vi "Read Data.vi"(8 "error in (no error)":errorcluster caption="entrée d'erreur (pas d'erreur)", 11 "Database Altyor en entrée":refnum<class "Database Altyor.lvclass">) -> (0 "error out":errorcluster caption="sortie d'erreur", 3 "Database Altyor en sortie":refnum<class "Database Altyor.lvclass">)   [LabVIEW 2020, in "Library Instrument & Equipement.lvlib" / "Library Database.lvlib" / "Database Altyor.lvclass"]
uses:
  Database Altyor.lvclass
  C:/Users/ngarcin/OneDrive - Altyor/Standard TB/Class/Database/Database drivers/Database Drivers.lvclass
  <vilib>/addons/database/_DB Variant To Data/Database Variant To Data.xnode
  Database Altyor.lvclass/Database Altyor.ctl
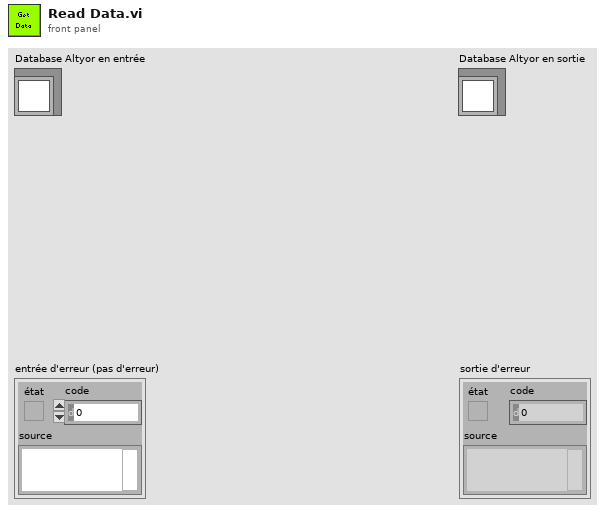
[diagram p1: front panel]
types:
  T1 = cluster{"idTest":u32, "CreationDate":string, "EndOfProduction":string, "OrderNumber":string, "Batch":string, "ProductName":string, "PartNumber":string, "SerialNumber":string, "Operator":string, "Result":string, "AdditionalInformation":string}[]
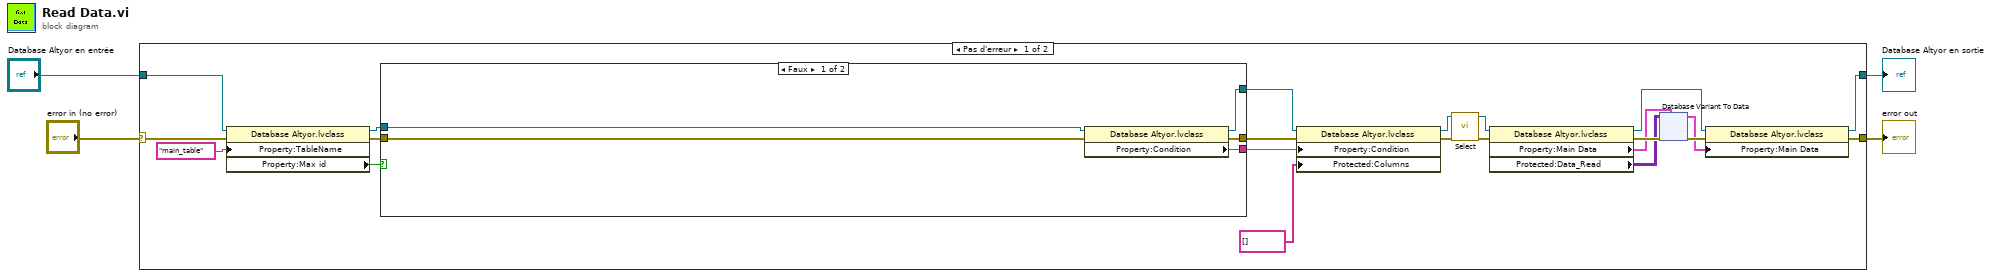
[diagram p0: block diagram]
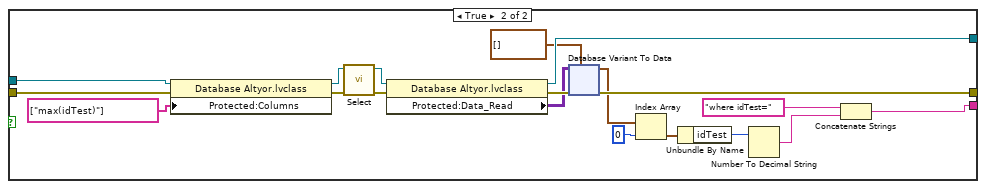
[diagram p2: hidden frame]
diagram:
  n1 = case shown="Pas d'erreur" "error in (no error)" {
    selector: "error in (no error)" -> [w13 w444]
    tunnel: [w22 w444] -> w3
    tunnel: [w20 w443] -> w1
    tunnel: "Database Altyor en entrée" -> [w14 w443]
    frame No Error {
      n2 = property class="Database Altyor.lvclass"(reference=w14, error in=w13, "Property:TableName"="main_table" ("TableName")) -> (reference out=w8:refnum<class "Database Altyor.lvclass">, error out=w10:errorcluster, "Property:Max id"=w11:bool)
      n3 = case shown="Faux" w11 {
        tunnel: w10 -> [w27 w50]
        tunnel: [w28 w42] -> w9
        tunnel: w8 -> [w31 w48]
        tunnel: [w30 w44] -> w7
        tunnel: [w29 w33] -> w5
        frame False {
          n4 = property class="Database Altyor.lvclass"(reference=w31, error in=w27) -> (reference out=w30:refnum<class "Database Altyor.lvclass">, error out=w28:errorcluster, "Property:Condition"=w29:string)
        }
        frame True {
          n5 = property class="Database Altyor.lvclass"(reference=w48, error in=w50, "Protected:Columns"=string[] ["max(idTest)"] ("Columns")) -> (reference out=w47:refnum<class "Database Altyor.lvclass">, error out=w49:errorcluster)
          n6 = call-dynamic "Select.vi"("error in (no error)"=w49, "Database Drivers en entrée"=w47) -> ("error out"=w46:errorcluster, "Database Drivers en sortie"=w45:refnum<class "Database Altyor.lvclass">)  [unwired: 8 in]
          n7 = property class="Database Altyor.lvclass"(reference=w45, error in=w46) -> (reference out=w44:refnum<class "Database Altyor.lvclass">, error out=w43:errorcluster, "Protected:Data_Read"=w41:variant[][])
          n8 = xnode "Database Variant To Data"("database variant"=w41, "error in (no error)"=w43, "type"=cluster{"idTest":u32}[] [] ("Main Data")) -> ("data"=w39:cluster{"idTest":u32}[], "error out"=w42:errorcluster)
          n9 = Index Array(array=w39, index=0 ("indice")) -> (element=w37:cluster{"idTest":u32})
          n10 = Unbundle By Name(w37) -> ("idTest"=w35:u32)
          n11 = Number To Decimal String(number=w35) -> (decimal integer string=w34:string)  [unwired: 1 in]
          n12 = Concatenate Strings("where idTest=" ("chaîne"), w34) -> (w33:string)
        }
      }
      n13 = property class="Database Altyor.lvclass"(reference=w7, error in=w9, "Property:Condition"=w5, "Protected:Columns"=string[] [] ("Columns")) -> (reference out=w23:refnum<class "Database Altyor.lvclass">, error out=w24:errorcluster)
      n14 = call-dynamic "Select.vi"("error in (no error)"=w24, "Database Drivers en entrée"=w23) -> ("error out"=w25:errorcluster, "Database Drivers en sortie"=w26:refnum<class "Database Altyor.lvclass">)  [unwired: 8 in]
      n15 = property class="Database Altyor.lvclass"(reference=w26, error in=w25) -> (reference out=w21:refnum<class "Database Altyor.lvclass">, error out=w19:errorcluster, "Property:Main Data"=w16:T1, "Protected:Data_Read"=w17:variant[][])
      n16 = xnode "Database Variant To Data"("database variant"=w17, "error in (no error)"=w19, "type"=w16) -> ("data"=w15:T1, "error out"=w18:errorcluster)
      n17 = property class="Database Altyor.lvclass"(reference=w21, error in=w18, "Property:Main Data"=w15) -> (reference out=w20:refnum<class "Database Altyor.lvclass">, error out=w22:errorcluster)
    }
    frame Error {
    }
  }
  "error out" <- w3
  "Database Altyor en sortie" <- w1
